vi "Check Paths.vi"(8 "Path Disabled Ref":refnum<vi>[](array[refnum]), 10 "Chuck Control ref in":T1, 11 "Glue Pathways":T3=[{"HDI Slot "=0, "Stamp Slot"=0, "Glue Slot"=0, "Weight Slot"=0, "BBM Slot"=0}, {"HDI Slot "=1, "Stamp Slot"=1, "Glue Slot"=1, "Weight Slot"=1, "BBM Slot"=1}, {"HDI Slot "=2, "Stamp Slot"=2, "Glue Slot"=2, "Weight Slot"=2, "BBM Slot"=2}, {"HDI Slot "=3, "Stamp Slot"=3, "Glue Slot"=3, "Weight Slot"=3, "BBM Slot"=3}] {"BBM Slot" items=["Slot 1", "Slot 2", "Slot 3", "Slot 4"]; "Weight Slot" items=["Slot 1", "Slot 2", "Slot 3", "Slot 4"]; "Glue Slot" items=["Slot 1", "Slot 2", "Slot 3", "Slot 4"]; "Stamp Slot" items=["Slot 1", "Slot 2", "Slot 3", "Slot 4"]; "HDI Slot" items=["Slot 1", "Slot 2", "Slot 3", "Slot 4"]}) -> (3 "Active Paths":T2=[TRUE, TRUE, TRUE, TRUE])   [LabVIEW 2017]
uses:
  UI typedefs/Glue Paths.ctl
  UI typedefs/Glue Path.ctl
  UI typedefs/Active Paths.ctl
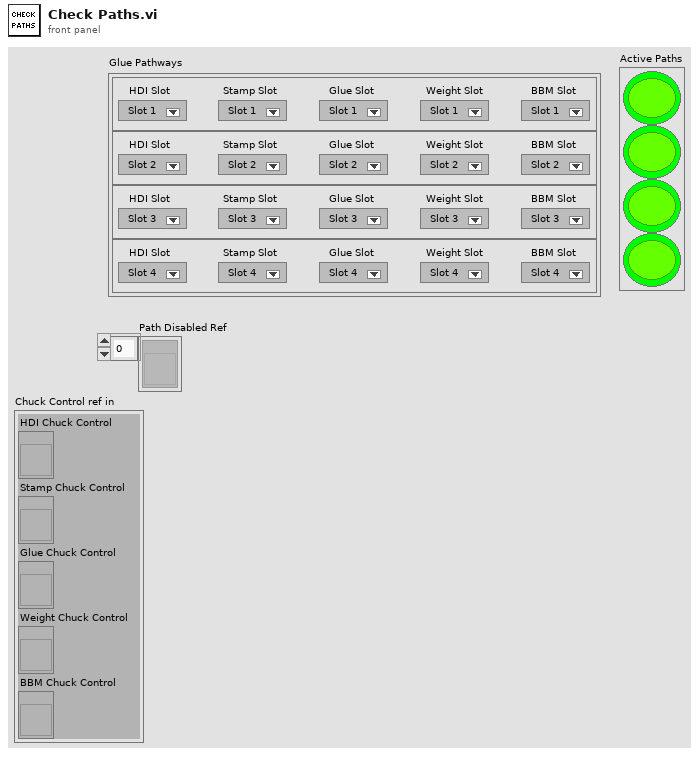
[diagram p1: front panel]
types:
  T1 = cluster{"HDI Chuck Control":refnum<vi>, "Stamp Chuck Control":refnum<vi>, "Glue Chuck Control":refnum<vi>, "Weight Chuck Control":refnum<vi>, "BBM Chuck Control":refnum<vi>}
  T2 = typedef "Active Paths.ctl" = bool[]
  T3 = typedef "Glue Paths.ctl" = T4[]
  T4 = typedef "Glue Path.ctl" = cluster{"HDI Slot ":i32, "Stamp Slot":i32, "Glue Slot":i32, "Weight Slot":i32, "BBM Slot":i32}
  T5 = typedef "HDI Chuck Control.ctl" = cluster{"Slot 1":T6, "Slot 2":T6, "Slot 3":T6, "Slot 4":T6}
  T6 = typedef "HDI Slot Control.ctl" = cluster{"Populated?":bool, "Identification:":string}
  T7 = typedef "Stamp Chuck Control.ctl" = cluster{"Slot 1":T8, "Slot 2":T8, "Slot 3":T8, "Slot 4":T8}
  T8 = typedef "Stamp Slot Control.ctl" = cluster{"Populated?":bool, "Stamp Type":T9}
  T9 = typedef "Stamp Type.ctl" = enum16{"Stamp 1", "Stamp 2", "Stamp 3", "Stamp 4", "Stamp 5", "Stamp 6", "Stamp 7", "Stamp 8"}
  T10 = typedef "Glue Chuck Control.ctl" = cluster{"Slot 1":T11, "Slot 2":T11, "Slot 3":T11, "Slot 4":T11}
  T11 = typedef "Glue Slot Control.ctl" = cluster{"Populated?":bool}
  T12 = typedef "Weight Chuck Control.ctl" = cluster{"Slot 1":T13, "Slot 2":T13, "Slot 3":T13, "Slot 4":T13}
  T13 = typedef "Weight Slot Control.ctl" = cluster{"Populated?":bool, "Weight Type":T14}
  T14 = typedef "Weight Type.ctl" = enum16{"Weight 1", "Weight 2", "Weight 3", "Weight 4", "Weight 5", "Weight 6", "Weight 7", "Weight 8", "Weight 9", "Weight 10", "Weight 11", "Weight 12", "Weight 13", "Weight 14", "Weight 15", "Weight 16"}
  T15 = typedef "BM Slot Control.ctl" = cluster{"Populated?":bool, "Identification:":string}
  T16 = cluster{"Slot 1":T15, "Slot 2":T15, "Slot 3":T15, "Slot 4":T15}
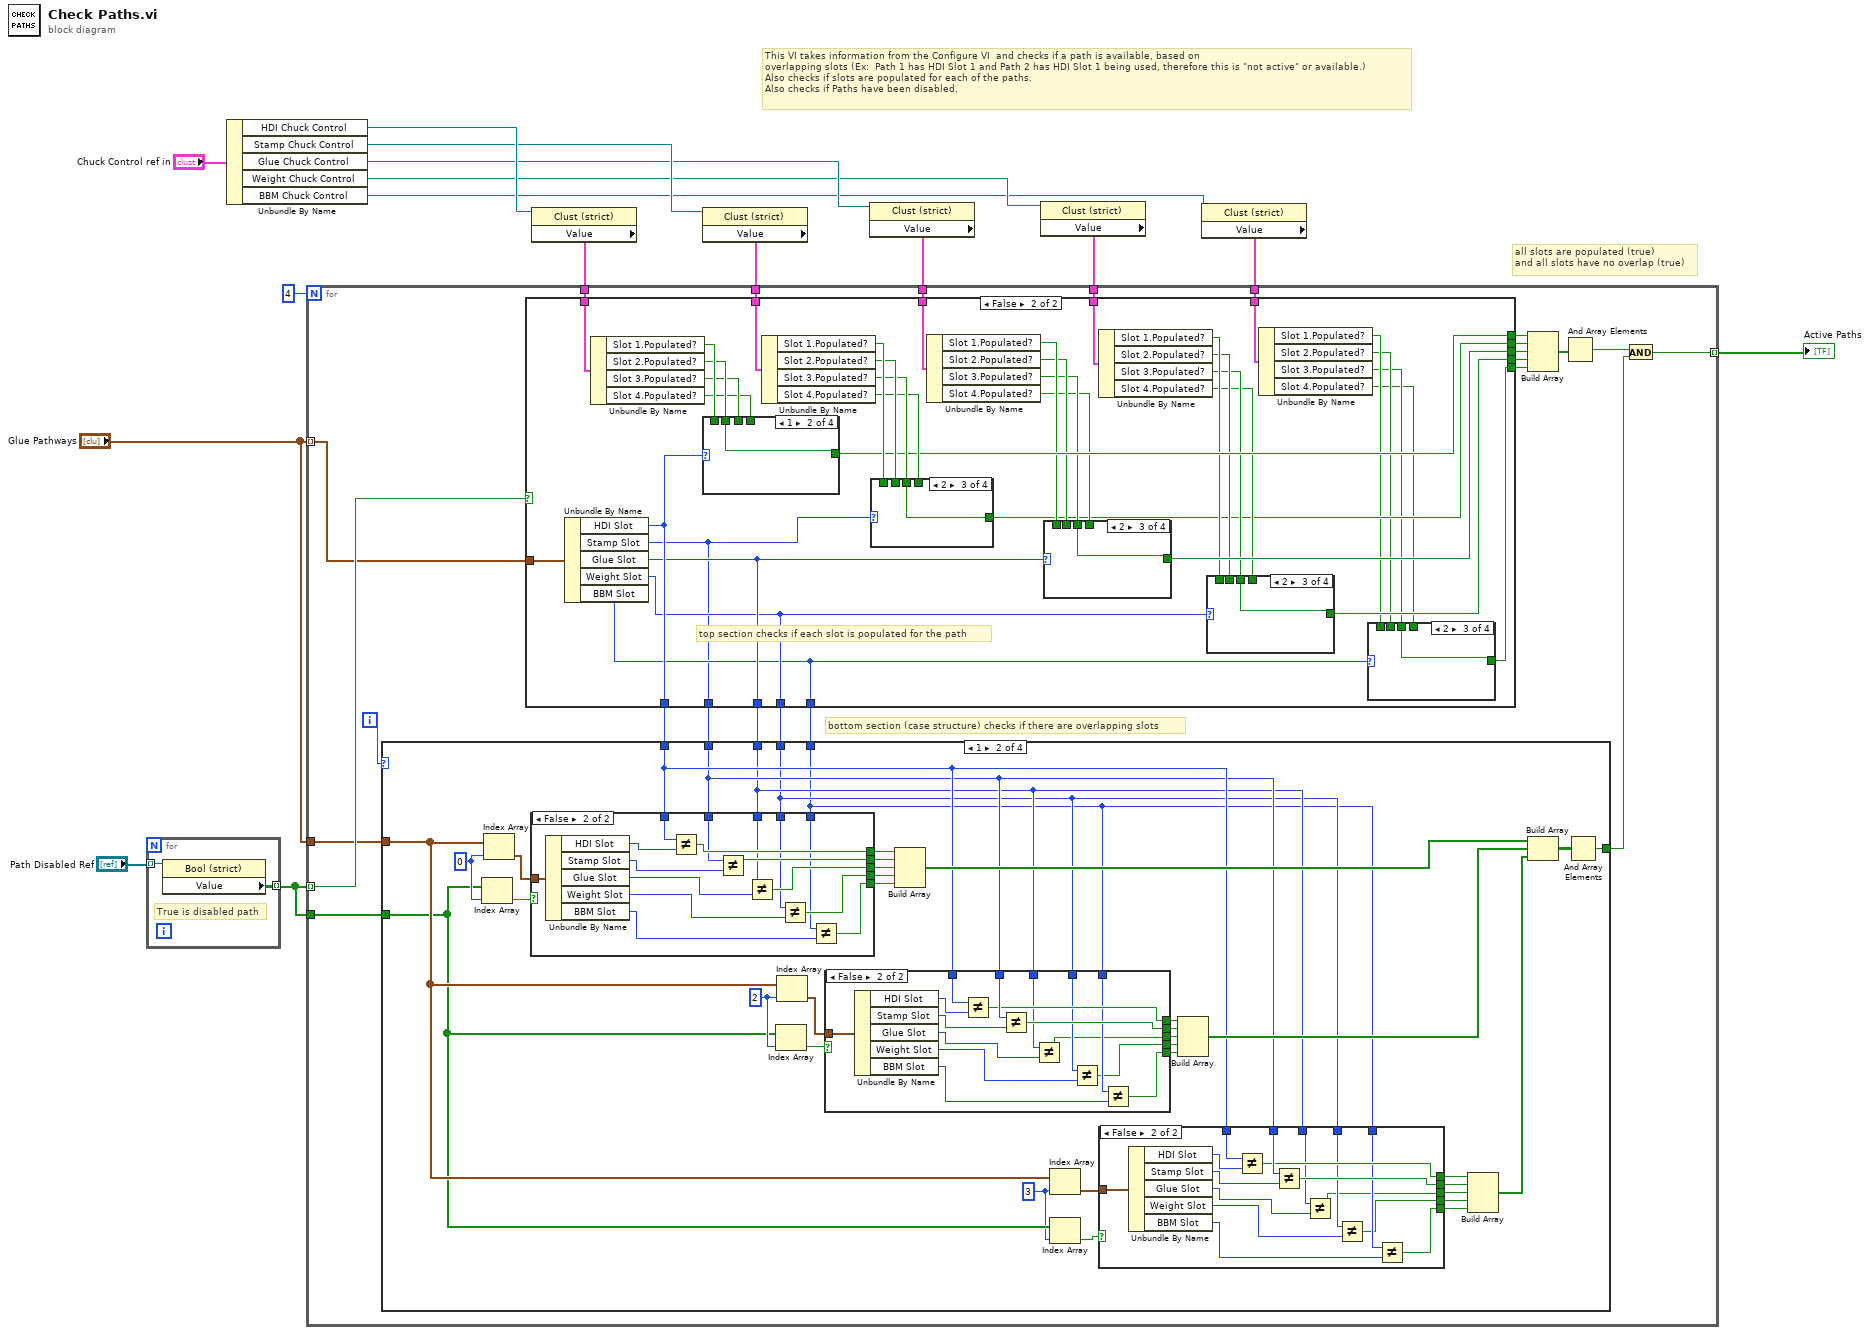
[diagram p0: block diagram]
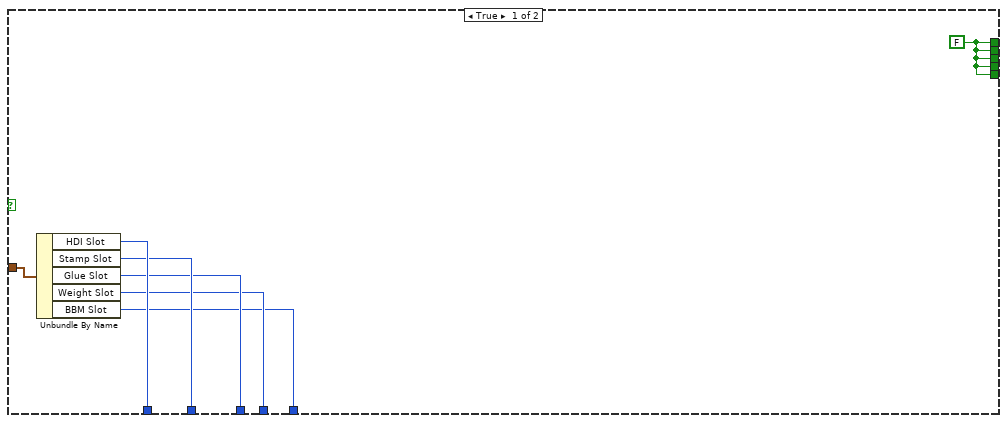
[diagram p2: hidden frame]
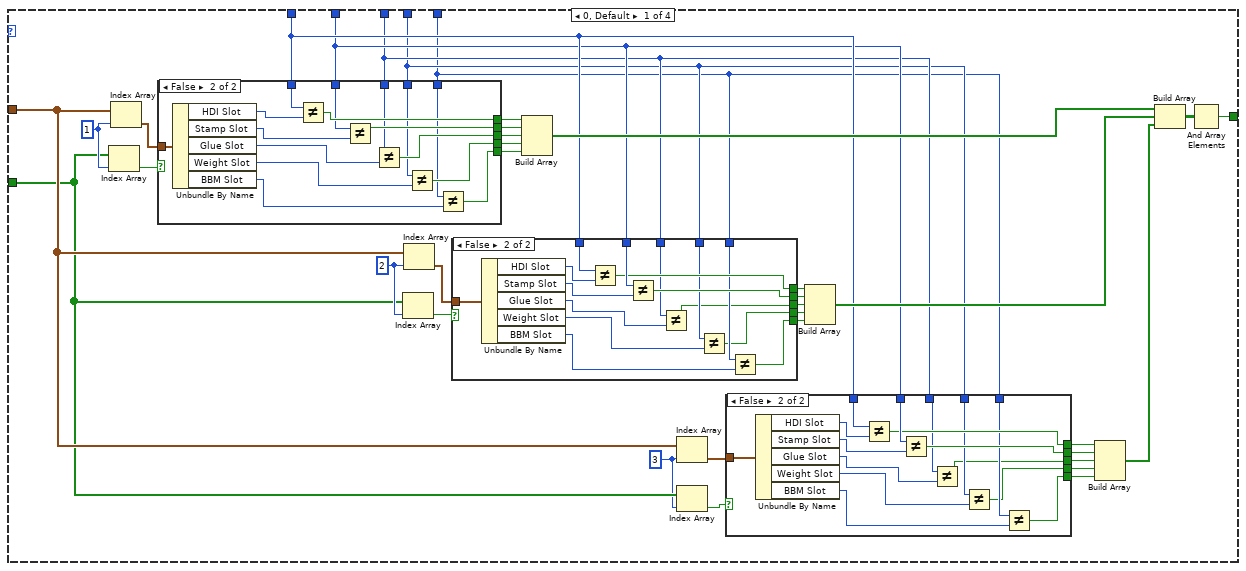
[diagram p18: hidden frame]
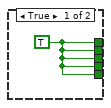
[diagram p19: hidden frame]
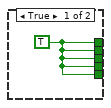
[diagram p20: hidden frame]
diagram:
  # "all slots are populated (true)\nand all slots have no overlap (true)"
  # "This VI takes information from the Configure VI  and checks if a path is available, based on\noverlapping slots (Ex:  Path 1 has HDI Slot 1 and Path 2 has HDI Slot 1 being used, therefore this is \"not active\" or available.)\nAlso checks if slots are populated for each of the paths.\nAlso checks if Paths have been disabled."
  n1 = for {
    tunnel: "Path Disabled Ref" -> [w18] mode=indexing
    tunnel: [w17] -> w2 mode=indexing
    # "True is disabled path"
    n2 = property class="Bool (strict)"(reference=w18) -> ("Value"=w17:bool)  [unwired: 1 in, 2 out]
  }
  n3 = Unbundle By Name("Chuck Control ref in") -> ("HDI Chuck Control"=w15:refnum<vi>, "Stamp Chuck Control"=w12:refnum<vi>, "Glue Chuck Control"=w10:refnum<vi>, "Weight Chuck Control"=w8:refnum<vi>, "BBM Chuck Control"=w7:refnum<vi>)
  n4 = property class="Clust (strict)"(reference=w15) -> ("Value"=w14:T5)  [unwired: 1 in, 2 out]
  n5 = property class="Clust (strict)"(reference=w12) -> ("Value"=w13:T7)  [unwired: 1 in, 2 out]
  n6 = property class="Clust (strict)"(reference=w10) -> ("Value"=w11:T10)  [unwired: 1 in, 2 out]
  n7 = property class="Clust (strict)"(reference=w8) -> ("Value"=w9:T12)  [unwired: 1 in, 2 out]
  n8 = property class="Clust (strict)"(reference=w7) -> ("Value"=w6:T16)  [unwired: 1 in, 2 out]
  n9 = for {
    N: 4 -> [_]
    tunnel: "Glue Pathways" -> [w21] mode=indexing
    tunnel: [w30] -> w4 mode=indexing
    tunnel: w14 -> [w28]
    tunnel: w13 -> [w27]
    tunnel: w11 -> [w26]
    tunnel: w9 -> [w25]
    tunnel: w6 -> [w24]
    tunnel: w2 -> [w22] mode=indexing
    tunnel: "Glue Pathways" -> [w20]
    tunnel: w2 -> [w19]
    i -> [w23]
    # "bottom section (case structure) checks if there are overlapping slots"
    n10 = case shown="False" w22 {
      tunnel: [w49 w77] -> w42
      tunnel: [w49 w76] -> w40
      tunnel: [w49 w67] -> w39
      tunnel: [w49 w66] -> w38
      tunnel: [w49 w65] -> w37
      tunnel: [w47 w60] -> w36
      tunnel: [w45 w59] -> w35
      tunnel: [w44 w58] -> w34
      tunnel: [w43 w57] -> w33
      tunnel: w21 -> [w48 w56]
      tunnel: [w46 w55] -> w29
      tunnel: w28 -> [_ w54]
      tunnel: w27 -> [_ w53]
      tunnel: w26 -> [_ w52]
      tunnel: w25 -> [_ w51]
      tunnel: w24 -> [_ w50]
      frame True {
        w49 = FALSE ("Populated?")
        n11 = Unbundle By Name(w48) -> ("HDI Slot"=w47:i32, "Stamp Slot"=w46:i32, "Glue Slot"=w45:i32, "Weight Slot"=w44:i32, "BBM Slot"=w43:i32)
      }
      frame False {
        # "top section checks if each slot is populated for the path"
        n12 = Unbundle By Name(w56) -> ("HDI Slot"=w60:i32, "Stamp Slot"=w55:i32, "Glue Slot"=w59:i32, "Weight Slot"=w58:i32, "BBM Slot"=w57:i32)
        n13 = Unbundle By Name(w54) -> ("Slot 1.Populated?"=w85:bool, "Slot 2.Populated?"=w84:bool, "Slot 3.Populated?"=w83:bool, "Slot 4.Populated?"=w82:bool)
        n14 = case shown="1" w60 {
          tunnel: w85 -> [w102 _ _ _]
          tunnel: [w102 w103 w104 w105] -> w77
          tunnel: w84 -> [_ w103 _ _]
          tunnel: w83 -> [_ _ w104 _]
          tunnel: w82 -> [_ _ _ w105]
          frame 0, Default {
          }
          frame 1 {
          }
          frame 2 {
          }
          frame 3 {
          }
        }
        n15 = Unbundle By Name(w53) -> ("Slot 1.Populated?"=w81:bool, "Slot 2.Populated?"=w80:bool, "Slot 3.Populated?"=w79:bool, "Slot 4.Populated?"=w78:bool)
        n16 = case shown="2" w55 {
          tunnel: [w98 w99 w100 w101] -> w65
          tunnel: w81 -> [w98 _ _ _]
          tunnel: w79 -> [_ _ w100 _]
          tunnel: w80 -> [_ w99 _ _]
          tunnel: w78 -> [_ _ _ w101]
          frame 0, Default {
          }
          frame 1 {
          }
          frame 2 {
          }
          frame 3 {
          }
        }
        n17 = Unbundle By Name(w52) -> ("Slot 1.Populated?"=w75:bool, "Slot 2.Populated?"=w74:bool, "Slot 3.Populated?"=w73:bool, "Slot 4.Populated?"=w72:bool)
        n18 = case shown="2" w59 {
          tunnel: [w94 w95 w96 w97] -> w76
          tunnel: w75 -> [w94 _ _ _]
          tunnel: w74 -> [_ w95 _ _]
          tunnel: w73 -> [_ _ w96 _]
          tunnel: w72 -> [_ _ _ w97]
          frame 0, Default {
          }
          frame 1 {
          }
          frame 2 {
          }
          frame 3 {
          }
        }
        n19 = Unbundle By Name(w51) -> ("Slot 1.Populated?"=w71:bool, "Slot 2.Populated?"=w70:bool, "Slot 3.Populated?"=w69:bool, "Slot 4.Populated?"=w68:bool)
        n20 = case shown="2" w58 {
          tunnel: [w90 w91 w92 w93] -> w67
          tunnel: w71 -> [w90 _ _ _]
          tunnel: w70 -> [_ w91 _ _]
          tunnel: w69 -> [_ _ w92 _]
          tunnel: w68 -> [_ _ _ w93]
          frame 0, Default {
          }
          frame 1 {
          }
          frame 2 {
          }
          frame 3 {
          }
        }
        n21 = Unbundle By Name(w50) -> ("Slot 1.Populated?"=w64:bool, "Slot 2.Populated?"=w63:bool, "Slot 3.Populated?"=w62:bool, "Slot 4.Populated?"=w61:bool)
        n22 = case shown="2" w57 {
          tunnel: [w86 w87 w88 w89] -> w66
          tunnel: w64 -> [w86 _ _ _]
          tunnel: w63 -> [_ w87 _ _]
          tunnel: w62 -> [_ _ w88 _]
          tunnel: w61 -> [_ _ _ w89]
          frame 0, Default {
          }
          frame 1 {
          }
          frame 2 {
          }
          frame 3 {
          }
        }
      }
    }
    n23 = case shown="1" w23 {
      tunnel: w36 -> [w115 w202 w289 w376]
      tunnel: w29 -> [w114 w201 w288 w375]
      tunnel: w35 -> [w113 w200 w287 w374]
      tunnel: w34 -> [w112 w199 w286 w373]
      tunnel: w33 -> [w106 w193 w280 w367]
      tunnel: [w135 w222 w309 w396] -> w31
      tunnel: w20 -> [w134 w221 w308 w395]
      tunnel: w19 -> [w117 w204 w291 w378]
      frame 0, Default {
        w116 = 3 ("index")
        w126 = 2 ("index")
        w133 = 1 ("index")
        n24 = Index Array(array=w117, index=w133) -> (element=w132:bool)
        n25 = Index Array(array=w134, index=w133) -> (element=w141:T4)
        n26 = case shown="False" w132 {
          tunnel: w141 -> [_ w192]
          tunnel: [w176 w189] -> w131
          tunnel: [w176 w186] -> w130
          tunnel: [w176 w183] -> w129
          tunnel: [w176 w180] -> w128
          tunnel: [w176 w177] -> w127
          tunnel: w115 -> [_ w191]
          tunnel: w114 -> [_ w187]
          tunnel: w113 -> [_ w184]
          tunnel: w112 -> [_ w182]
          tunnel: w106 -> [_ w178]
          frame True {
            w176 = TRUE
          }
          frame False {
            n27 = Unbundle By Name(w192) -> ("HDI Slot"=w190:i32, "Stamp Slot"=w188:i32, "Glue Slot"=w185:i32, "Weight Slot"=w181:i32, "BBM Slot"=w179:i32)
            n28 = Not Equal?(x=w191, y=w190) -> (x != y?=w189:bool)
            n29 = Not Equal?(x=w187, y=w188) -> (x != y?=w186:bool)
            n30 = Not Equal?(x=w184, y=w185) -> (x != y?=w183:bool)
            n31 = Not Equal?(x=w182, y=w181) -> (x != y?=w180:bool)
            n32 = Not Equal?(x=w178, y=w179) -> (x != y?=w177:bool)
          }
        }
        n33 = Index Array(array=w117, index=w126) -> (element=w120:bool)
        n34 = Index Array(array=w134, index=w126) -> (element=w140:T4)
        n35 = case shown="False" w120 {
          tunnel: w140 -> [_ w175]
          tunnel: [w159 w170] -> w125
          tunnel: [w159 w169] -> w124
          tunnel: [w159 w162] -> w123
          tunnel: [w159 w161] -> w122
          tunnel: [w159 w160] -> w121
          tunnel: w115 -> [_ w173]
          tunnel: w114 -> [_ w172]
          tunnel: w113 -> [_ w168]
          tunnel: w112 -> [_ w166]
          tunnel: w106 -> [_ w163]
          frame True {
            w159 = TRUE
          }
          frame False {
            n36 = Unbundle By Name(w175) -> ("HDI Slot"=w174:i32, "Stamp Slot"=w171:i32, "Glue Slot"=w167:i32, "Weight Slot"=w165:i32, "BBM Slot"=w164:i32)
            n37 = Not Equal?(x=w173, y=w174) -> (x != y?=w170:bool)
            n38 = Not Equal?(x=w172, y=w171) -> (x != y?=w169:bool)
            n39 = Not Equal?(x=w168, y=w167) -> (x != y?=w162:bool)
            n40 = Not Equal?(x=w166, y=w165) -> (x != y?=w161:bool)
            n41 = Not Equal?(x=w163, y=w164) -> (x != y?=w160:bool)
          }
        }
        n42 = Build Array(w131, w130, w129, w128, w127) -> (w139:bool[])
        n43 = Index Array(array=w134, index=w116) -> (element=w119:T4)
        n44 = Index Array(array=w117, index=w116) -> (element=w118:bool)
        n45 = case shown="False" w118 {
          tunnel: w119 -> [_ w158]
          tunnel: [w142 w153] -> w111
          tunnel: [w142 w152] -> w110
          tunnel: [w142 w145] -> w109
          tunnel: [w142 w144] -> w108
          tunnel: [w142 w143] -> w107
          tunnel: w115 -> [_ w156]
          tunnel: w114 -> [_ w155]
          tunnel: w113 -> [_ w151]
          tunnel: w112 -> [_ w149]
          tunnel: w106 -> [_ w146]
          frame True {
            w142 = TRUE
          }
          frame False {
            n46 = Unbundle By Name(w158) -> ("HDI Slot"=w157:i32, "Stamp Slot"=w154:i32, "Glue Slot"=w150:i32, "Weight Slot"=w148:i32, "BBM Slot"=w147:i32)
            n47 = Not Equal?(x=w156, y=w157) -> (x != y?=w153:bool)
            n48 = Not Equal?(x=w155, y=w154) -> (x != y?=w152:bool)
            n49 = Not Equal?(x=w151, y=w150) -> (x != y?=w145:bool)
            n50 = Not Equal?(x=w149, y=w148) -> (x != y?=w144:bool)
            n51 = Not Equal?(x=w146, y=w147) -> (x != y?=w143:bool)
          }
        }
        n52 = Build Array(w125, w124, w123, w122, w121) -> (w138:bool[])
        n53 = Build Array(w111, w110, w109, w108, w107) -> (w137:bool[])
        n54 = Build Array(w139, w138, w137) -> (w136:bool[][])
        n55 = And Array Elements(Boolean array=w136) -> (logical AND=w135:bool)
      }
      frame 1 {
        w203 = 3 ("index")
        w213 = 2 ("index")
        w220 = 0 ("index")
        n56 = Index Array(array=w204, index=w220) -> (element=w219:bool)
        n57 = Index Array(array=w221, index=w220) -> (element=w228:T4)
        n58 = case shown="False" w219 {
          tunnel: w228 -> [_ w279]
          tunnel: [w263 w276] -> w218
          tunnel: [w263 w273] -> w217
          tunnel: [w263 w270] -> w216
          tunnel: [w263 w267] -> w215
          tunnel: [w263 w264] -> w214
          tunnel: w202 -> [_ w278]
          tunnel: w201 -> [_ w274]
          tunnel: w200 -> [_ w271]
          tunnel: w199 -> [_ w269]
          tunnel: w193 -> [_ w265]
          frame True {
            w263 = TRUE
          }
          frame False {
            n59 = Unbundle By Name(w279) -> ("HDI Slot"=w277:i32, "Stamp Slot"=w275:i32, "Glue Slot"=w272:i32, "Weight Slot"=w268:i32, "BBM Slot"=w266:i32)
            n60 = Not Equal?(x=w278, y=w277) -> (x != y?=w276:bool)
            n61 = Not Equal?(x=w274, y=w275) -> (x != y?=w273:bool)
            n62 = Not Equal?(x=w271, y=w272) -> (x != y?=w270:bool)
            n63 = Not Equal?(x=w269, y=w268) -> (x != y?=w267:bool)
            n64 = Not Equal?(x=w265, y=w266) -> (x != y?=w264:bool)
          }
        }
        n65 = Index Array(array=w204, index=w213) -> (element=w207:bool)
        n66 = Index Array(array=w221, index=w213) -> (element=w227:T4)
        n67 = case shown="False" w207 {
          tunnel: w227 -> [_ w262]
          tunnel: [w246 w257] -> w212
          tunnel: [w246 w256] -> w211
          tunnel: [w246 w249] -> w210
          tunnel: [w246 w248] -> w209
          tunnel: [w246 w247] -> w208
          tunnel: w202 -> [_ w260]
          tunnel: w201 -> [_ w259]
          tunnel: w200 -> [_ w255]
          tunnel: w199 -> [_ w253]
          tunnel: w193 -> [_ w250]
          frame True {
            w246 = TRUE
          }
          frame False {
            n68 = Unbundle By Name(w262) -> ("HDI Slot"=w261:i32, "Stamp Slot"=w258:i32, "Glue Slot"=w254:i32, "Weight Slot"=w252:i32, "BBM Slot"=w251:i32)
            n69 = Not Equal?(x=w260, y=w261) -> (x != y?=w257:bool)
            n70 = Not Equal?(x=w259, y=w258) -> (x != y?=w256:bool)
            n71 = Not Equal?(x=w255, y=w254) -> (x != y?=w249:bool)
            n72 = Not Equal?(x=w253, y=w252) -> (x != y?=w248:bool)
            n73 = Not Equal?(x=w250, y=w251) -> (x != y?=w247:bool)
          }
        }
        n74 = Build Array(w218, w217, w216, w215, w214) -> (w226:bool[])
        n75 = Index Array(array=w221, index=w203) -> (element=w206:T4)
        n76 = Index Array(array=w204, index=w203) -> (element=w205:bool)
        n77 = case shown="False" w205 {
          tunnel: w206 -> [_ w245]
          tunnel: [w229 w240] -> w198
          tunnel: [w229 w239] -> w197
          tunnel: [w229 w232] -> w196
          tunnel: [w229 w231] -> w195
          tunnel: [w229 w230] -> w194
          tunnel: w202 -> [_ w243]
          tunnel: w201 -> [_ w242]
          tunnel: w200 -> [_ w238]
          tunnel: w199 -> [_ w236]
          tunnel: w193 -> [_ w233]
          frame True {
            w229 = TRUE
          }
          frame False {
            n78 = Unbundle By Name(w245) -> ("HDI Slot"=w244:i32, "Stamp Slot"=w241:i32, "Glue Slot"=w237:i32, "Weight Slot"=w235:i32, "BBM Slot"=w234:i32)
            n79 = Not Equal?(x=w243, y=w244) -> (x != y?=w240:bool)
            n80 = Not Equal?(x=w242, y=w241) -> (x != y?=w239:bool)
            n81 = Not Equal?(x=w238, y=w237) -> (x != y?=w232:bool)
            n82 = Not Equal?(x=w236, y=w235) -> (x != y?=w231:bool)
            n83 = Not Equal?(x=w233, y=w234) -> (x != y?=w230:bool)
          }
        }
        n84 = Build Array(w212, w211, w210, w209, w208) -> (w225:bool[])
        n85 = Build Array(w198, w197, w196, w195, w194) -> (w224:bool[])
        n86 = Build Array(w226, w225, w224) -> (w223:bool[][])
        n87 = And Array Elements(Boolean array=w223) -> (logical AND=w222:bool)
      }
      frame 2 {
        w290 = 3 ("index")
        w300 = 1 ("index")
        w307 = 0 ("index")
        n88 = Index Array(array=w291, index=w307) -> (element=w306:bool)
        n89 = Index Array(array=w308, index=w307) -> (element=w315:T4)
        n90 = case shown="False" w306 {
          tunnel: w315 -> [_ w366]
          tunnel: [w350 w363] -> w305
          tunnel: [w350 w360] -> w304
          tunnel: [w350 w357] -> w303
          tunnel: [w350 w354] -> w302
          tunnel: [w350 w351] -> w301
          tunnel: w289 -> [_ w365]
          tunnel: w288 -> [_ w361]
          tunnel: w287 -> [_ w358]
          tunnel: w286 -> [_ w356]
          tunnel: w280 -> [_ w352]
          frame True {
            w350 = TRUE
          }
          frame False {
            n91 = Unbundle By Name(w366) -> ("HDI Slot"=w364:i32, "Stamp Slot"=w362:i32, "Glue Slot"=w359:i32, "Weight Slot"=w355:i32, "BBM Slot"=w353:i32)
            n92 = Not Equal?(x=w365, y=w364) -> (x != y?=w363:bool)
            n93 = Not Equal?(x=w361, y=w362) -> (x != y?=w360:bool)
            n94 = Not Equal?(x=w358, y=w359) -> (x != y?=w357:bool)
            n95 = Not Equal?(x=w356, y=w355) -> (x != y?=w354:bool)
            n96 = Not Equal?(x=w352, y=w353) -> (x != y?=w351:bool)
          }
        }
        n97 = Index Array(array=w291, index=w300) -> (element=w294:bool)
        n98 = Index Array(array=w308, index=w300) -> (element=w314:T4)
        n99 = case shown="False" w294 {
          tunnel: w314 -> [_ w349]
          tunnel: [w333 w344] -> w299
          tunnel: [w333 w343] -> w298
          tunnel: [w333 w336] -> w297
          tunnel: [w333 w335] -> w296
          tunnel: [w333 w334] -> w295
          tunnel: w289 -> [_ w347]
          tunnel: w288 -> [_ w346]
          tunnel: w287 -> [_ w342]
          tunnel: w286 -> [_ w340]
          tunnel: w280 -> [_ w337]
          frame True {
            w333 = TRUE
          }
          frame False {
            n100 = Unbundle By Name(w349) -> ("HDI Slot"=w348:i32, "Stamp Slot"=w345:i32, "Glue Slot"=w341:i32, "Weight Slot"=w339:i32, "BBM Slot"=w338:i32)
            n101 = Not Equal?(x=w347, y=w348) -> (x != y?=w344:bool)
            n102 = Not Equal?(x=w346, y=w345) -> (x != y?=w343:bool)
            n103 = Not Equal?(x=w342, y=w341) -> (x != y?=w336:bool)
            n104 = Not Equal?(x=w340, y=w339) -> (x != y?=w335:bool)
            n105 = Not Equal?(x=w337, y=w338) -> (x != y?=w334:bool)
          }
        }
        n106 = Build Array(w305, w304, w303, w302, w301) -> (w313:bool[])
        n107 = Index Array(array=w308, index=w290) -> (element=w293:T4)
        n108 = Index Array(array=w291, index=w290) -> (element=w292:bool)
        n109 = case shown="False" w292 {
          tunnel: w293 -> [_ w332]
          tunnel: [w316 w327] -> w285
          tunnel: [w316 w326] -> w284
          tunnel: [w316 w319] -> w283
          tunnel: [w316 w318] -> w282
          tunnel: [w316 w317] -> w281
          tunnel: w289 -> [_ w330]
          tunnel: w288 -> [_ w329]
          tunnel: w287 -> [_ w325]
          tunnel: w286 -> [_ w323]
          tunnel: w280 -> [_ w320]
          frame True {
            w316 = TRUE
          }
          frame False {
            n110 = Unbundle By Name(w332) -> ("HDI Slot"=w331:i32, "Stamp Slot"=w328:i32, "Glue Slot"=w324:i32, "Weight Slot"=w322:i32, "BBM Slot"=w321:i32)
            n111 = Not Equal?(x=w330, y=w331) -> (x != y?=w327:bool)
            n112 = Not Equal?(x=w329, y=w328) -> (x != y?=w326:bool)
            n113 = Not Equal?(x=w325, y=w324) -> (x != y?=w319:bool)
            n114 = Not Equal?(x=w323, y=w322) -> (x != y?=w318:bool)
            n115 = Not Equal?(x=w320, y=w321) -> (x != y?=w317:bool)
          }
        }
        n116 = Build Array(w299, w298, w297, w296, w295) -> (w312:bool[])
        n117 = Build Array(w285, w284, w283, w282, w281) -> (w311:bool[])
        n118 = Build Array(w313, w312, w311) -> (w310:bool[][])
        n119 = And Array Elements(Boolean array=w310) -> (logical AND=w309:bool)
      }
      frame 3 {
        w377 = 2 ("index")
        w387 = 1 ("index")
        w394 = 0 ("index")
        n120 = Index Array(array=w378, index=w394) -> (element=w393:bool)
        n121 = Index Array(array=w395, index=w394) -> (element=w402:T4)
        n122 = case shown="False" w393 {
          tunnel: w402 -> [_ w453]
          tunnel: [w437 w450] -> w392
          tunnel: [w437 w447] -> w391
          tunnel: [w437 w444] -> w390
          tunnel: [w437 w441] -> w389
          tunnel: [w437 w438] -> w388
          tunnel: w376 -> [_ w452]
          tunnel: w375 -> [_ w448]
          tunnel: w374 -> [_ w445]
          tunnel: w373 -> [_ w443]
          tunnel: w367 -> [_ w439]
          frame True {
            w437 = TRUE
          }
          frame False {
            n123 = Unbundle By Name(w453) -> ("HDI Slot"=w451:i32, "Stamp Slot"=w449:i32, "Glue Slot"=w446:i32, "Weight Slot"=w442:i32, "BBM Slot"=w440:i32)
            n124 = Not Equal?(x=w452, y=w451) -> (x != y?=w450:bool)
            n125 = Not Equal?(x=w448, y=w449) -> (x != y?=w447:bool)
            n126 = Not Equal?(x=w445, y=w446) -> (x != y?=w444:bool)
            n127 = Not Equal?(x=w443, y=w442) -> (x != y?=w441:bool)
            n128 = Not Equal?(x=w439, y=w440) -> (x != y?=w438:bool)
          }
        }
        n129 = Index Array(array=w378, index=w387) -> (element=w381:bool)
        n130 = Index Array(array=w395, index=w387) -> (element=w401:T4)
        n131 = case shown="False" w381 {
          tunnel: w401 -> [_ w436]
          tunnel: [w420 w431] -> w386
          tunnel: [w420 w430] -> w385
          tunnel: [w420 w423] -> w384
          tunnel: [w420 w422] -> w383
          tunnel: [w420 w421] -> w382
          tunnel: w376 -> [_ w434]
          tunnel: w375 -> [_ w433]
          tunnel: w374 -> [_ w429]
          tunnel: w373 -> [_ w427]
          tunnel: w367 -> [_ w424]
          frame True {
            w420 = TRUE
          }
          frame False {
            n132 = Unbundle By Name(w436) -> ("HDI Slot"=w435:i32, "Stamp Slot"=w432:i32, "Glue Slot"=w428:i32, "Weight Slot"=w426:i32, "BBM Slot"=w425:i32)
            n133 = Not Equal?(x=w434, y=w435) -> (x != y?=w431:bool)
            n134 = Not Equal?(x=w433, y=w432) -> (x != y?=w430:bool)
            n135 = Not Equal?(x=w429, y=w428) -> (x != y?=w423:bool)
            n136 = Not Equal?(x=w427, y=w426) -> (x != y?=w422:bool)
            n137 = Not Equal?(x=w424, y=w425) -> (x != y?=w421:bool)
          }
        }
        n138 = Build Array(w392, w391, w390, w389, w388) -> (w400:bool[])
        n139 = Index Array(array=w395, index=w377) -> (element=w380:T4)
        n140 = Index Array(array=w378, index=w377) -> (element=w379:bool)
        n141 = case shown="False" w379 {
          tunnel: w380 -> [_ w419]
          tunnel: [w403 w414] -> w372
          tunnel: [w403 w413] -> w371
          tunnel: [w403 w406] -> w370
          tunnel: [w403 w405] -> w369
          tunnel: [w403 w404] -> w368
          tunnel: w376 -> [_ w417]
          tunnel: w375 -> [_ w416]
          tunnel: w374 -> [_ w412]
          tunnel: w373 -> [_ w410]
          tunnel: w367 -> [_ w407]
          frame True {
            w403 = TRUE
          }
          frame False {
            n142 = Unbundle By Name(w419) -> ("HDI Slot"=w418:i32, "Stamp Slot"=w415:i32, "Glue Slot"=w411:i32, "Weight Slot"=w409:i32, "BBM Slot"=w408:i32)
            n143 = Not Equal?(x=w417, y=w418) -> (x != y?=w414:bool)
            n144 = Not Equal?(x=w416, y=w415) -> (x != y?=w413:bool)
            n145 = Not Equal?(x=w412, y=w411) -> (x != y?=w406:bool)
            n146 = Not Equal?(x=w410, y=w409) -> (x != y?=w405:bool)
            n147 = Not Equal?(x=w407, y=w408) -> (x != y?=w404:bool)
          }
        }
        n148 = Build Array(w386, w385, w384, w383, w382) -> (w399:bool[])
        n149 = Build Array(w372, w371, w370, w369, w368) -> (w398:bool[])
        n150 = Build Array(w400, w399, w398) -> (w397:bool[][])
        n151 = And Array Elements(Boolean array=w397) -> (logical AND=w396:bool)
      }
    }
    n152 = Build Array(w42, w37, w40, w39, w38) -> (w41:bool[])
    n153 = And Array Elements(Boolean array=w41) -> (logical AND=w32:bool)
    n154 = And(x=w32, y=w31) -> (x .and. y?=w30:bool)
  }
  "Active Paths" <- w4
